vi "Tag Not Found.vi"(7 "caller name":string, 8 "error in (no error)":errorcluster, 10 "found?":bool, 11 "Tag Name":string) -> (0 "error out":errorcluster)   [LabVIEW 2016, in "CVT.lvlib" / "Current Value Table.lvlib"]
doc: "This VI throws an error if a tag cannot be located."
uses:
  <vilib>/NI/Current Value Table/Current Value Table.lvlib
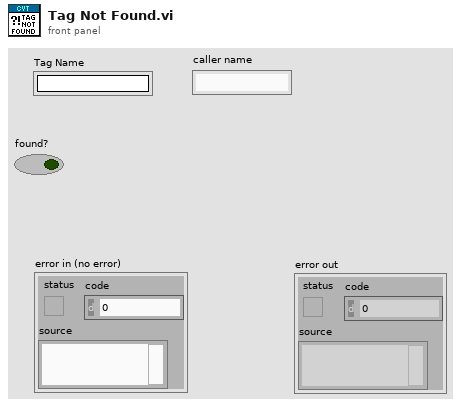
[diagram p1: front panel]
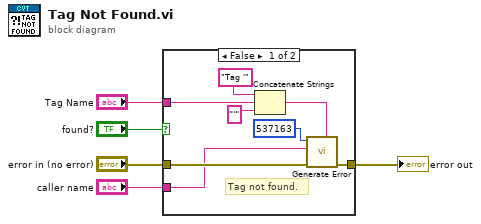
[diagram p0: block diagram]
diagram:
  n1 = case shown="False" "found?" {
    tunnel: "error in (no error)" -> [w9 w14]
    tunnel: [w8 w14] -> w4
    tunnel: "Tag Name" -> [w7 _]
    tunnel: "caller name" -> [w6 _]
    frame False {
      # "Tag not found."
      n2 = Concatenate Strings("Tag '" ("string"), w7, "'" ("string")) -> (w10:string)
      n3 = call <vilib>:"Generate Error.vi"("<append> (\"\")"=w10, "error in"=w9, "caller name"=w6, "code"=537163) -> ("error out"=w8:errorcluster)  [unwired: 7 in]
    }
    frame True {
    }
  }
  "error out" <- w4
